vi "PAQ_Retrieve_latest_DB_data.vi"(8 "error in (no error)":errorcluster, 11 "FAMM-Attributes in":T1={"FAMM_PAQ_Layers"=0, "FAMM_PAQ_resolution"=0.0, "PAQ_TAGs"=[], "WAQ_TAGs"=[], "EAQ_TAGs"=[], "All_TAGs"=[], "PAQtagProps"=[], "WAQtagProps"=[], "EAQtagProps"=[], "DBAL_class"=refnum, "PAQ_memory"=[], "PAQupdates"=[], "FAMM_Size"={"other"=0, "1day"=0, "1week"=0}, "DatabaseFileExtention"="", "DatabaseSaveRate"=0.0, "Database_path"=path "G:/Sgraph_database", "DBAL-Queue"=refnum, "OS_name"="undefined", "ini-file"="", "data-retention(days)"=0.0} {"FAMM_Size"."1week" format="%.0p"; "FAMM_Size"."1day" format="%.0p"; "FAMM_Size"."other" format="%.0p"; "EAQtagProps"."TagFunc" format="%08x"; "EAQtagProps"."RangeL" format="%.2f"; "EAQtagProps"."RangeH" format="%.2f"; "WAQtagProps"."TagFunc" format="%08x"; "WAQtagProps"."RangeL" format="%.2f"; "WAQtagProps"."RangeH" format="%.2f"; "PAQtagProps"."TagFunc" format="%08x"; "PAQtagProps"."RangeL" format="%.2f"; "PAQtagProps"."RangeH" format="%.2f"; "FAMM_PAQ_resolution" format="%.1p"}) -> (0 "error out":errorcluster, 3 "FAMM-Attributes out":T1={"FAMM_PAQ_Layers"=0, "FAMM_PAQ_resolution"=0.0, "PAQ_TAGs"=[], "WAQ_TAGs"=[], "EAQ_TAGs"=[], "All_TAGs"=[], "PAQtagProps"=[], "WAQtagProps"=[], "EAQtagProps"=[], "DBAL_class"=refnum, "PAQ_memory"=[], "PAQupdates"=[], "FAMM_Size"={"other"=0, "1day"=0, "1week"=0}, "DatabaseFileExtention"="", "DatabaseSaveRate"=0.0, "Database_path"=path "G:/Sgraph_database", "DBAL-Queue"=refnum, "OS_name"="undefined", "ini-file"="", "data-retention(days)"=0.0} {"FAMM_Size"."1week" format="%.0p"; "FAMM_Size"."1day" format="%.0p"; "FAMM_Size"."other" format="%.0p"; "EAQtagProps"."TagFunc" format="%08x"; "EAQtagProps"."RangeL" format="%.2f"; "EAQtagProps"."RangeH" format="%.2f"; "WAQtagProps"."TagFunc" format="%08x"; "WAQtagProps"."RangeL" format="%.2f"; "WAQtagProps"."RangeH" format="%.2f"; "PAQtagProps"."TagFunc" format="%08x"; "PAQtagProps"."RangeL" format="%.2f"; "PAQtagProps"."RangeH" format="%.2f"; "FAMM_PAQ_resolution" format="%.1p"})   [LabVIEW 2020, in "Sgraph_lib_V1.lvlib" / "FAMM.lvclass"]
uses:
  FAMM.lvclass
  controls/FAMM-attributes.ctl
  Common/controls/typedef_com_TagProp.ctl
  DBAL/DBAL.lvclass
  PAQ-memory.lvclass
  DBAL/controls/DBAL_Command.ctl
  DBAL/controls/DBAL-commands.ctl
  DBAL/controls/DBAL_FetchLatestFrom.ctl
  PAQ-memory.lvclass/PAQ-memory.ctl
  Builds/Sgraph_lib_V1.lvlib
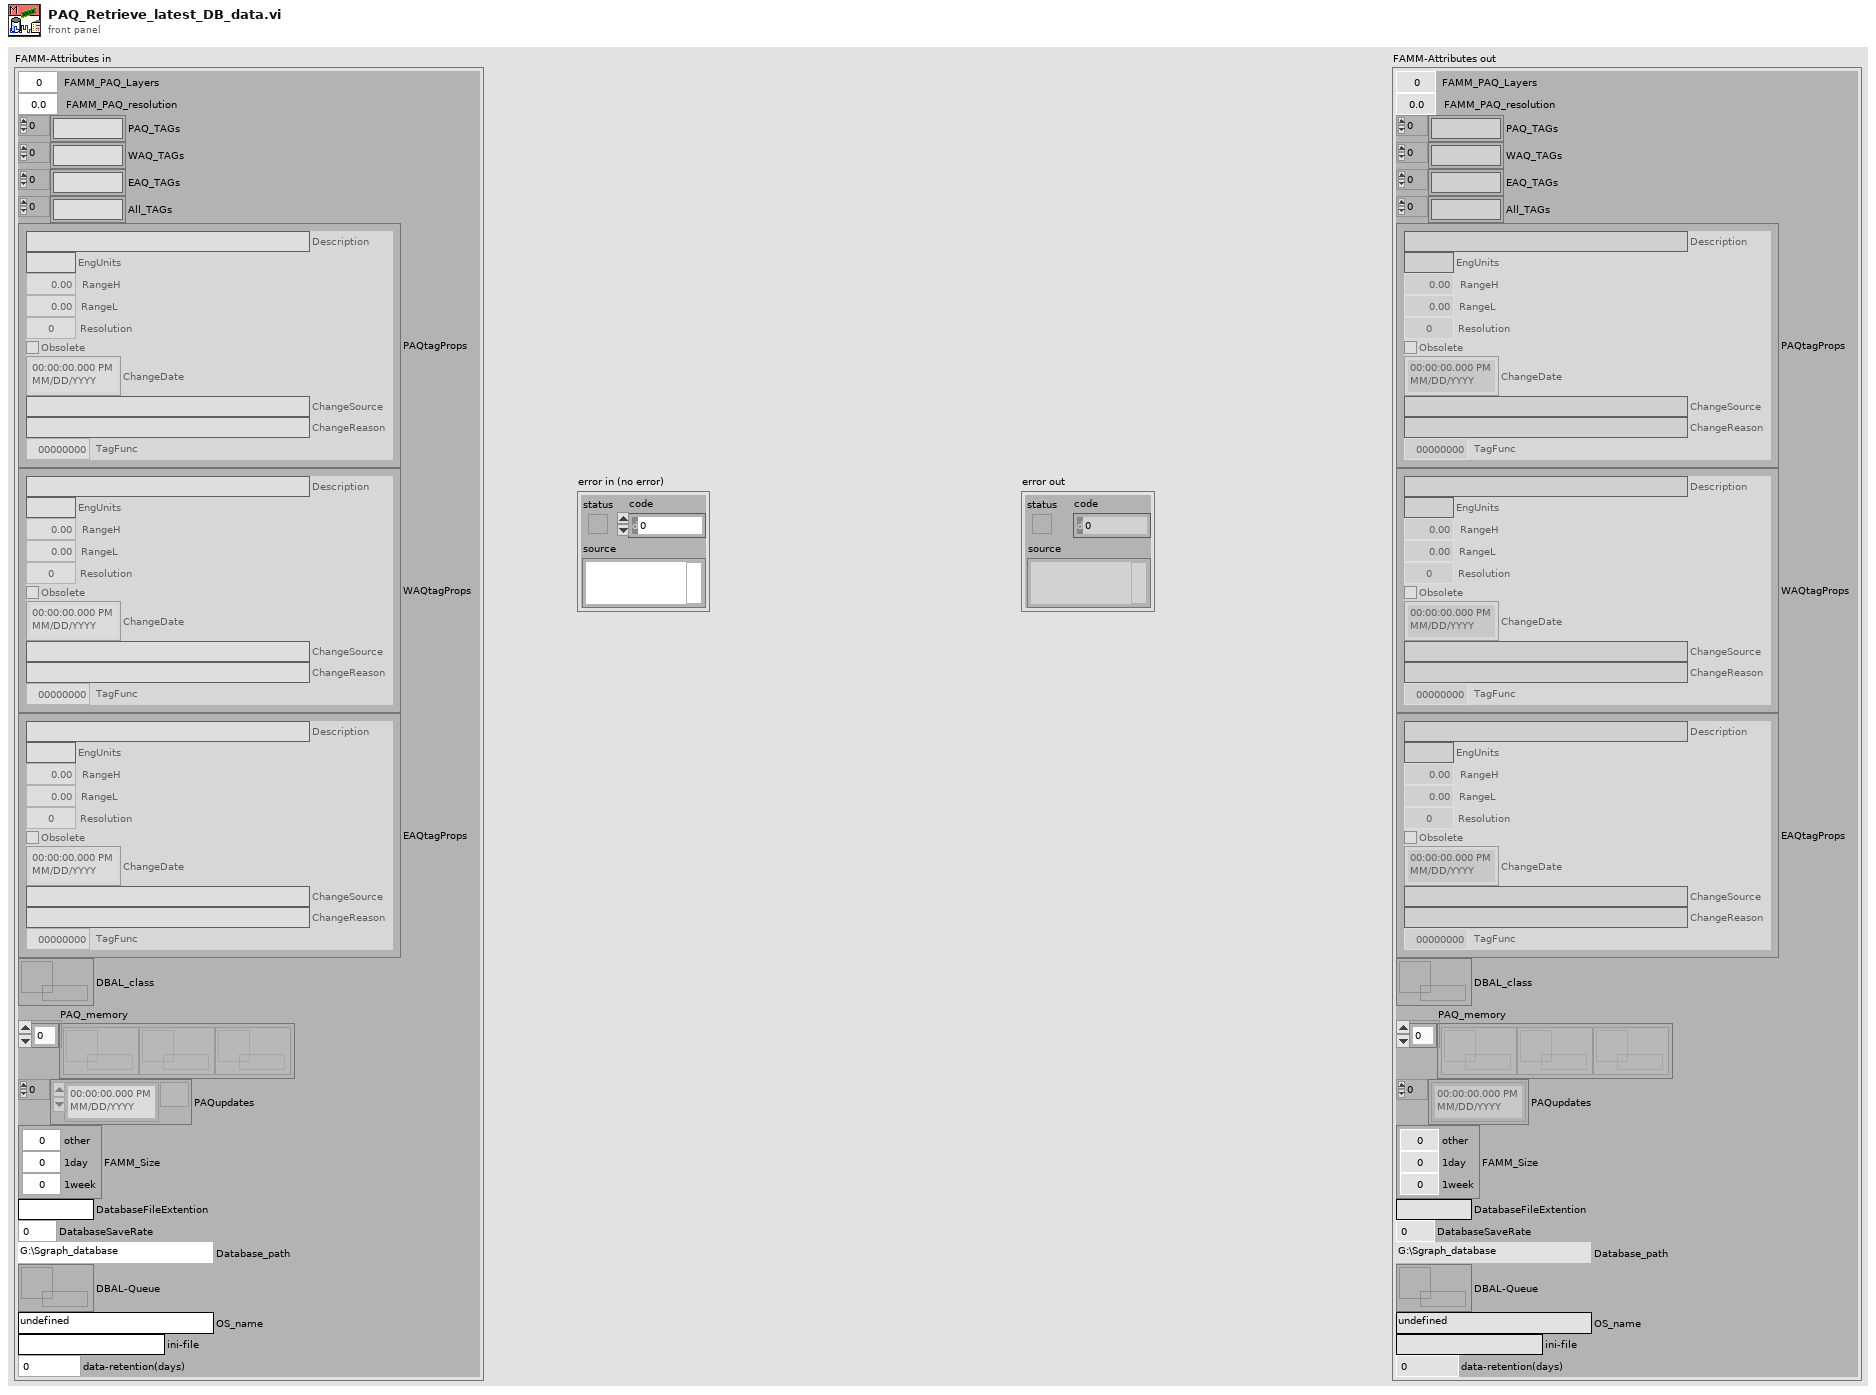
[diagram p1: front panel]
types:
  T1 = typedef "Sgraph_lib_V1.lvlib/FAMM.lvclass/FAMM-attributes.ctl" = cluster{"FAMM_PAQ_Layers":i32, "FAMM_PAQ_resolution":dbl, "PAQ_TAGs":string[], "WAQ_TAGs":string[], "EAQ_TAGs":string[], "All_TAGs":string[], "PAQtagProps":T2[], "WAQtagProps":T2[], "EAQtagProps":T2[], "DBAL_class":refnum<data-value>, "PAQ_memory":refnum<data-value>[], "PAQupdates":timestamp[], "FAMM_Size":cluster{"other":i32, "1day":i32, "1week":i32}, "DatabaseFileExtention":string, "DatabaseSaveRate":dbl, "Database_path":path, "DBAL-Queue":refnum<queue>, "OS_name":string, "ini-file":string, "data-retention(days)":dbl}
  T2 = typedef "Sgraph_lib_V1.lvlib/typedef_com_TagProp.ctl" = cluster{"Description":string, "EngUnits":string, "RangeH":dbl, "RangeL":dbl, "Resolution":i32, "Obsolete":bool, "ChangeDate":timestamp, "ChangeSource":string, "ChangeReason":string, "TagFunc":u32}
  T3 = typedef "Sgraph_lib_V1.lvlib/DBAL.lvclass/DBAL_FetchLatestFrom.ctl" = cluster{"Samples-Quantity":i32, "TableName":string, "PAQ_TAGs":string[]}
  T4 = typedef "Sgraph_lib_V1.lvlib/DBAL-BIN.lvclass/BINdata.ctl" = cluster{"time":dbl[], "TagsData":cluster{"data":dbl[], "max":dbl[], "min":dbl[], "status":u32[]}[]}
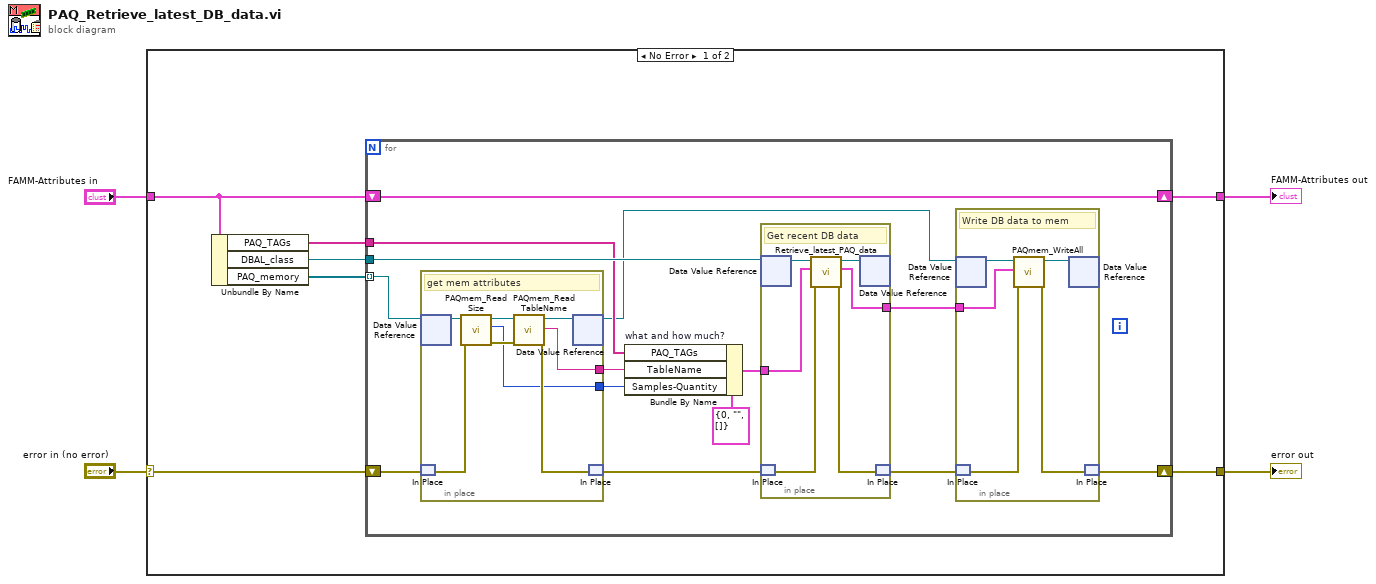
[diagram p0: block diagram]
diagram:
  n1 = case shown="No Error" "error in (no error)" {
    selector: "error in (no error)" -> [w9 w46]
    tunnel: [w8 w46] -> w3
    tunnel: [w7 w45] -> w1
    tunnel: "FAMM-Attributes in" -> [w10 w45]
    frame No Error {
      n2 = Unbundle By Name(w10) -> ("PAQ_TAGs"=w5:string[], "DBAL_class"=w6:refnum<data-value>, "PAQ_memory"=w11:refnum<data-value>[])
      n3 = for {
        tunnel: w11 -> [w22] mode=indexing
        shift-right: [w13] -> w8
        shift-left: w9 -> [w21]
        shift-right: [w25] -> w7
        shift-left: w10 -> [w25]
        tunnel: w6 -> [w17]
        tunnel: w5 -> [w16]
        n4 = in-place {
          in-place-border: [w32] -> w19
          in-place-border: [w31] -> w18
          # "get mem attributes"
          n5 = in-place-dvr #1(w22) -> (w38:refnum<class "PAQ-memory.lvclass">)  [unwired: 1 out]
          n6 = in-place-match #2(w21) -> (w35:errorcluster)
          n7 = call "PAQmem_Read Size.vi"("error in (no error)"=w35, "PAQ-memory in"=w38) -> ("error out"=w34:errorcluster, "Size"=w31:i32, "PAQ-memory out"=w37:refnum<class "PAQ-memory.lvclass">)  [unwired: 7 in]
          n8 = call "PAQmem_Read TableName.vi"("error in (no error)"=w34, "PAQ-memory in"=w37) -> ("error out"=w33:errorcluster, "TableName"=w32:string, "PAQ-memory out"=w36:refnum<class "PAQ-memory.lvclass">)  [unwired: 7 in]
          n9 = in-place-dvr #1(w36) -> (w15:refnum<data-value>)  [unwired: 1 out]
          n10 = in-place-match #2(w33) -> (w20:errorcluster)
        }
        n11 = Bundle By Name "what and how much?"(cluster=T3 {"Samples-Quantity"=0, "TableName"="", "PAQ_TAGs"=[]} ("FetchLatestDefinition"), "PAQ_TAGs"=w16, "TableName"=w19, "Samples-Quantity"=w18) -> (w24:T3)
        n12 = in-place {
          in-place-border: w24 -> [w40]
          in-place-border: [w39] -> w12
          # "Get recent DB data"
          n13 = in-place-dvr #3(w17) -> (w44:refnum<class "DBAL.lvclass">)  [unwired: 1 out]
          n14 = in-place-match #4(w20) -> (w42:errorcluster)
          n15 = call-dynamic "Retrieve_latest_PAQ_data.vi"("error in (no error)"=w42, "FetchLatestDefinition"=w40, "DBAL in"=w44) -> ("error out"=w41:errorcluster, "BinHistData"=w39:T4, "DBAL out"=w43:refnum<class "DBAL.lvclass">)  [unwired: 6 in]
          n16 = in-place-dvr #3(w43) -> ()  [unwired: 2 out]
          n17 = in-place-match #4(w41) -> (w14:errorcluster)
        }
        n18 = in-place {
          in-place-border: w12 -> [w26]
          # "Write DB data to mem"
          n19 = in-place-dvr #5(w15) -> (w30:refnum<class "PAQ-memory.lvclass">)  [unwired: 1 out]
          n20 = in-place-match #6(w14) -> (w28:errorcluster)
          n21 = call "PAQmem_WriteAll.vi"("error in (no error)"=w28, "BinHistData"=w26, "PAQ-memory in"=w30) -> ("error out"=w27:errorcluster, "PAQ-memory out"=w29:refnum<class "PAQ-memory.lvclass">)  [unwired: 7 in]
          n22 = in-place-dvr #5(w29) -> ()  [unwired: 2 out]
          n23 = in-place-match #6(w27) -> (w13:errorcluster)
        }
      }
    }
    frame Error {
    }
  }
  "error out" <- w3
  "FAMM-Attributes out" <- w1
